vi "10.Evd.4_Ask.4.vi"() -> ()   [LabVIEW 2025]
panel:
  in  "Cancel Button":bool
  out "String 3":string
  in  "Password":string
  in  "Username":string
  in  "OK Button":bool
  out "String 2":string
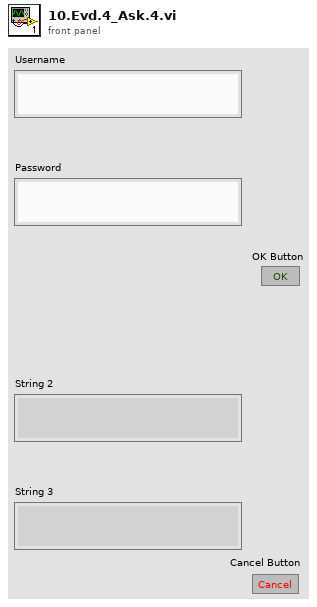
[diagram p1: front panel]
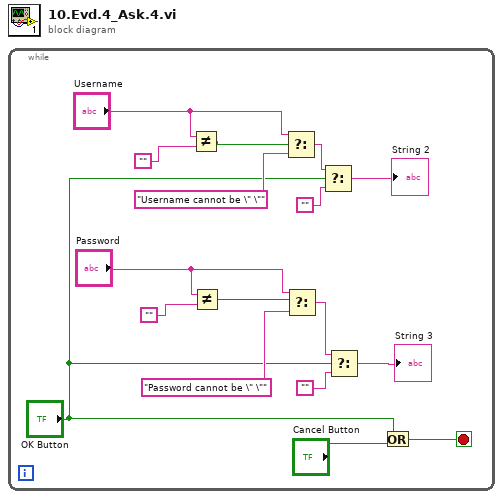
[diagram p0: block diagram]
diagram:
  n1 = while {
    stop <- w13 stop-if-true
    n2 = Not Equal?(x="Username", y="") -> (x != y?=w9:bool)
    n3 = Not Equal?(x="Password", y="") -> (x != y?=w5:bool)
    n4 = Select(t="Username", s=w9, f="Username cannot be \" \"") -> (s? t:f=w8:string)
    n5 = Select(t="Password", s=w5, f="Password cannot be \" \"") -> (s? t:f=w4:string)
    n6 = Select(t=w8, s="OK Button", f="") -> (s? t:f=→"String 2":string)
    n7 = Select(t=w4, s="OK Button", f="") -> (s? t:f=→"String 3":string)
    n8 = Or(x="OK Button", y="Cancel Button") -> (x .or. y?=w13:bool)
  }
